vi "Tracker_v2.2_test_acq_comms.vi"() -> ()   [LabVIEW 2018]
uses:
  <vilib>/Platform/TimedLoop/XDataNode/timing_clust.ctl
  <vilib>/Platform/TimedLoop/XDataNode/nitl_modes.ctl
  <vilib>/Platform/TimedLoop/XDataNode/wakeup.ctl
  <vilib>/Platform/TimedLoop/scheduler/LVUserAPI/_suppVIs/Create_1kHz_TSource.vi
  <vilib>/platform/TimedLoop/XDataNode/XDataNode.xnode
  <vilib>/Analysis/NI_AALBase.lvlib
  <vilib>/Platform/TimedLoop/XDataNode/XDNodeRunTimeDep.lvlib
panel:
  out "x/y":dbl format="%#_6f"
  out "# elements in queue":i32
  out "standard deviation":dbl format="%.3f"
  out "mean":dbl format="%.3f"
  out "mean 2":dbl format="%.5f"
  out "Instrument OK?":bool
  in  "Stop Button":bool
  out "DEC output cluster":T1
  in  "Play/Pause":bool
  in  "VISA resource name in":refnum<visa-resource-name>="ASRL3::INSTR"
  out "Waveform Chart":T2(graph)
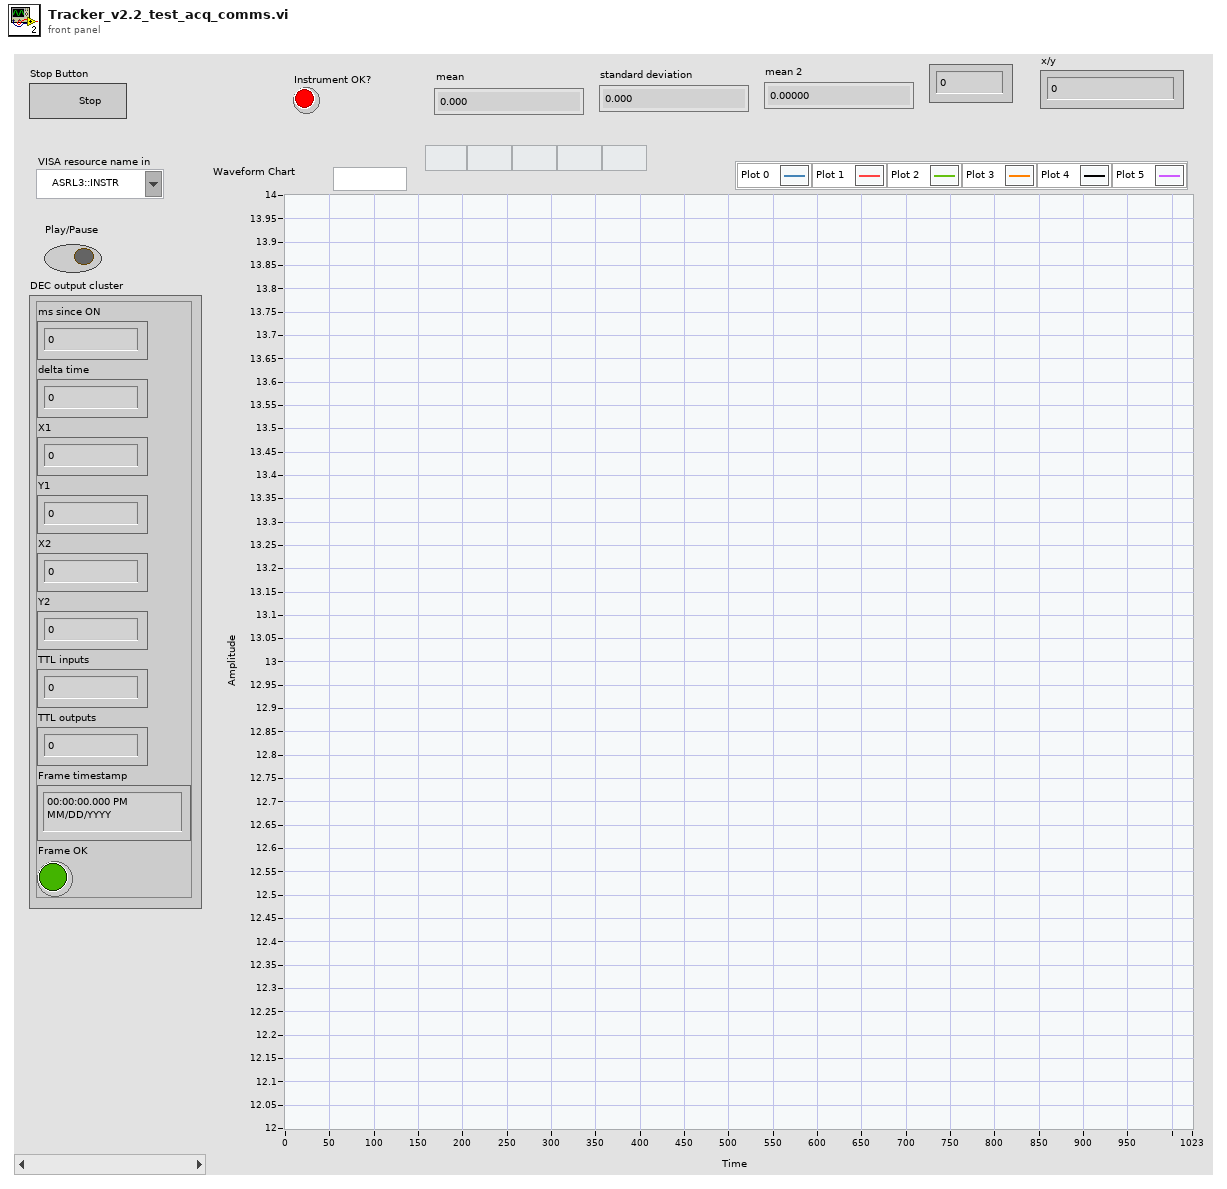
[diagram p1: front panel]
types:
  T1 = cluster{"ms since ON":u32, "delta time":u32, "X1":sgl, "Y1":sgl, "X2":sgl, "Y2":sgl, "TTL inputs":u8, "TTL outputs":u8, "Frame timestamp":timestamp, "Frame OK":bool}
  T2 = cluster{ext, "mean":dbl, "delta time":u32, "mean":dbl, i16}
  T3 = cluster{"Read buffer":string, "Timestamp":timestamp}
  T4 = typedef "CTL_Data_flow_control_cluster.ctl" = cluster{"Data acquisition status":refnum<notifier>, "Play/Pause status":refnum<notifier>, "Complete stop":refnum<notifier>, "Temp file ready for processing":refnum<notifier>, "Has been recorded":refnum<notifier>, "Recording now":refnum<notifier>, "Path to the latest complete temp file":refnum<notifier>, "(Final) Data file is saved":refnum<notifier>, "Data loaded":refnum<notifier>}
  T5 = typedef "XDNodeRunTimeDep.lvlib/timing_clust.ctl" = cluster{"Expected End [f-1]":u64, "Actual End [f-1]":u64, "Finished Late? [f-1]":bool, "Expected End [i-1]":u64, "Actual End [i-1]":u64, "Finished Late? [i-1]":bool, "Expected Start [i]":u64, "Actual Start [i]":u64, "Expected Start [f]":u64, "Actual Start [f]":u64, "Source Name":string, "Structure Name":string, "Period":i64, "Deadline":i64, "Offset":i64, "Start":i64, "Priority":i32, "Timeout":i32, "Mode":T6, "Wakeup Reason":T7, "Error":errorcluster, "Source Type":string, "Secondary Source Type":string, "Global End Time":u64, "Global Start Time":u64, "Frame Duration":u64, "Iteration Duration":u64, "Assigned CPU":i32, "I/O Scan Engine Mode":u32}
  T6 = typedef "XDNodeRunTimeDep.lvlib/nitl_modes.ctl" = enum32{"No Change", "Process missed periods, maintain original phase", "Discard missed periods, maintain original phase", "Process missed periods, ignore original phase", "Discard missed periods, ignore original phase"}
  T7 = typedef "XDNodeRunTimeDep.lvlib/wakeup.ctl" = enum32{"Normal", "Aborted", "Asynchronous wakeup", "Timing source error", "Timed loop error", "Timeout"}
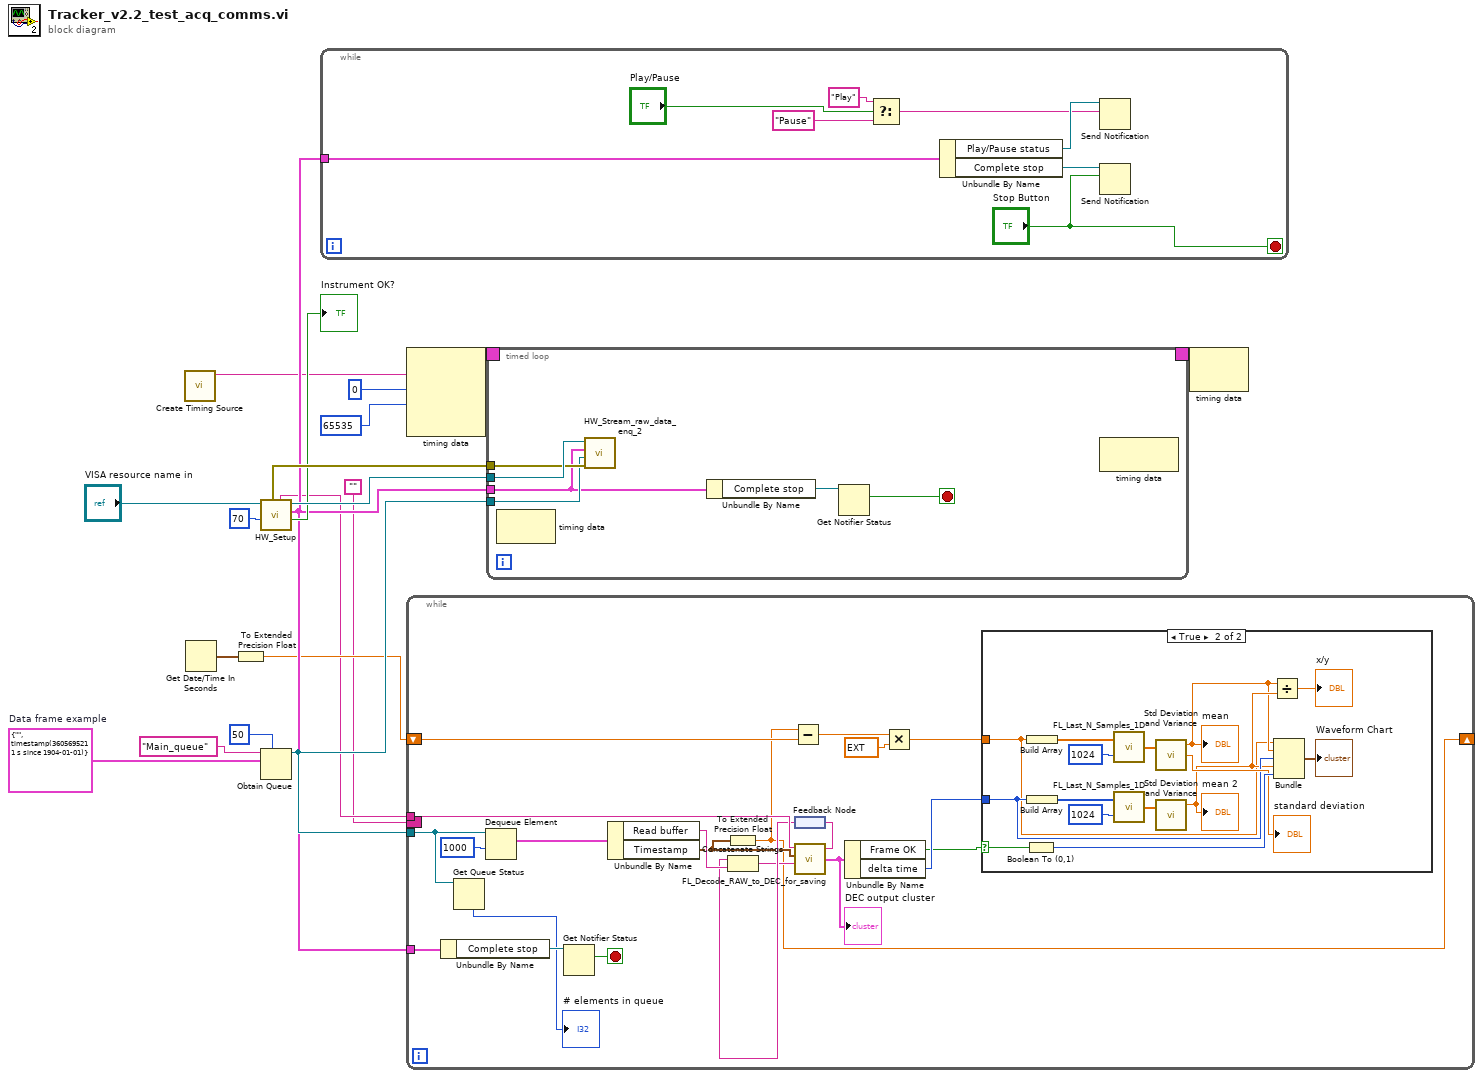
[diagram p0: block diagram]
diagram:
  w15 = T3 {"Read buffer"="", "Timestamp"=timestamp(3605695211.9516535 s since 1904-01-01)}  # Data frame example
  n1 = call-poly <vilib>:"Create Timing Source.vi"() -> ("name (out)"=w5:string)  [unwired: 10 in, 1 out]
  n2 = Get Date/Time In Seconds() -> (seconds since 1Jan1904=w9:timestamp)
  n3 = To Extended Precision Float(1:w9) -> (0:w8:ext)
  n4 = call "HW_Setup.vi"("Traget FPS"=70, "VISA resource name in"="VISA resource name in") -> ("Instrument OK?"=→"Instrument OK?":bool, "Data flow controls"=w10:T4, "VISA resource name out"=w18:refnum<visa-resource-name>, "Sensor board size"=w2:string, "error out"=w16:errorcluster)  [unwired: 2 in, 3 out]
  n5 = Obtain Queue(max queue size (-1, unlimited)=50, name (unnamed)="Main_queue", element data type=w15) -> (queue out=w11:refnum<queue>)  [unwired: 2 in, 2 out]
  n6 = while {
    tunnel: w10 -> [w27]
    stop <- "Stop Button" stop-if-true
    n7 = Select(t="Play", s="Play/Pause", f="Pause") -> (s? t:f=w24:string)
    n8 = Unbundle By Name(w27) -> ("Play/Pause status"=w26:refnum<notifier>, "Complete stop"=w20:refnum<notifier>)
    n9 = Send Notification(notification=w24, notifier=w26) -> ()  [unwired: 1 in, 2 out]
    n10 = Send Notification(notification="Stop Button", notifier=w20) -> ()  [unwired: 1 in, 2 out]
  }
  n11 = node-c288(w5, i64 0 ("Period"), 65535 ("Priority")) -> (w7:T5)  [unwired: 1 in]
  n12 = while {
    tunnel: w11 -> [w40]
    tunnel: w10 -> [w47]
    shift-right: [w28] -> _
    shift-left: w8 -> [w41]
    tunnel: w2 -> [w38]
    border: "" -> [_]
    stop <- w46 stop-if-true
    n13 = Unbundle By Name(w47) -> ("Complete stop"=w48:refnum<notifier>)
    n14 = Get Queue Status(queue=w40) -> (# elements in queue=→"# elements in queue":i32)  [unwired: 2 in, 7 out]
    n15 = Dequeue Element(queue=w40, timeout in ms (-1)=1000) -> (element=w44:T3)  [unwired: 1 in, 3 out]
    n16 = Get Notifier Status(notifier=w48) -> (current notification=w46:bool)  [unwired: 1 in, 4 out]
    n17 = Unbundle By Name(w44) -> ("Read buffer"=w37:string, "Timestamp"=w32:timestamp)
    n18 = To Extended Precision Float(1:w32) -> (0:w28:ext)
    n19 = Subtract(x=w28, y=w41) -> (x-y=w43:ext)
    n20 = feedback #1() -> (w36:string)
    n21 = Concatenate Strings(w36, w37) -> (w35:string)
    n22 = call "FL_Decode_RAW_to_DEC_for_saving.vi"("Sensor board size"=w38, "Input timestamp"=w32, "Input string"=w35) -> ("Output string leftover"=w33:string, "DEC output cluster"=w34:T1)  [unwired: 3 in, 1 out]
    "DEC output cluster" <- w34
    n23 = feedback-in #1(w33) -> ()
    n24 = Unbundle By Name(w34) -> ("Frame OK"=w30:bool, "delta time"=w31:u32)
    n25 = Multiply(x=w43, y=ext 1000.0) -> (x*y=w29:ext)
    n26 = case shown="True" w30 {
      selector: w30 -> [_ w54]
      tunnel: w31 -> [_ w57]
      tunnel: w29 -> [_ w49]
      frame False {
      }
      frame True {
        n27 = Boolean To (0,1)(Boolean=w54) -> (0, 1=w62:i16)
        n28 = Build Array(w49) -> (w59:ext[])
        n29 = Build Array(w57) -> (w61:u32[])
        n30 = call "FL_Last_N_Samples_1D.vi"("BufferLengthSamples"=u32 1024, "Input Array"=w59) -> ("Output Array"=w51:dbl[])
        n31 = call "FL_Last_N_Samples_1D.vi"("BufferLengthSamples"=u32 1024, "Input Array"=w61) -> ("Output Array"=w63:dbl[])
        n32 = call <vilib>:"Std Deviation and Variance.vi"("X"=w51) -> ("mean"=w50:dbl, "standard deviation"=→"standard deviation":dbl)  [unwired: 1 in, 1 out]
        "mean" <- w50
        n33 = call <vilib>:"Std Deviation and Variance.vi"("X"=w63) -> ("mean"=w53:dbl)  [unwired: 1 in, 2 out]
        "mean 2" <- w53
        n34 = Divide(x=w50, y=w53) -> (x/y=→"x/y":dbl)
        n35 = Bundle(w49, "mean"=w50, "delta time"=w57, "mean"=w53, w62) -> (→"Waveform Chart":T2)  [unwired: 1 in]
      }
    }
  }
  n36 = timed-loop {
    tunnel: w18 -> [w69]
    tunnel: w10 -> [w66]
    tunnel: w16 -> [w68]
    tunnel: w11 -> [w67]
    timing: w7 -> [_]
    timing-out: [_] -> w6
    stop <- w64 stop-if-true
    n37 = node-c288() -> ()  [unwired: 1 in, 1 out]
    n38 = call "HW_Stream_raw_data_enq_2.vi"("error in"=w68, "Queue in"=w67, "Data flow controls in"=w66, "VISA resource name in"=w69) -> ()  [unwired: 4 in, 4 out]
    n39 = Unbundle By Name(w66) -> ("Complete stop"=w65:refnum<notifier>)
    n40 = Get Notifier Status(notifier=w65) -> (current notification=w64:bool)  [unwired: 1 in, 4 out]
    n41 = node-c288() -> ()  [unwired: 1 in, 1 out]
  }
  n42 = node-c288(w6) -> ()  [unwired: 1 out]
